vi "DAQ.Create.vi"(8 "error in":errorcluster, 11 "Instrument.DAQ":refnum<class "Instrument.DAQ.lvclass">) -> (0 "error out":errorcluster, 3 "Instrument.DAQ":refnum<class "Instrument.DAQ.lvclass">)   [LabVIEW 2019, in "Instrument.Lockin.lvlib" / "Instrument.DAQ.lvclass"]
uses:
  Instrument.DAQ.lvclass
  Instrument.DAQ.lvclass/Instrument.DAQ.ctl
  DAQmx/DAQmx.lvclass
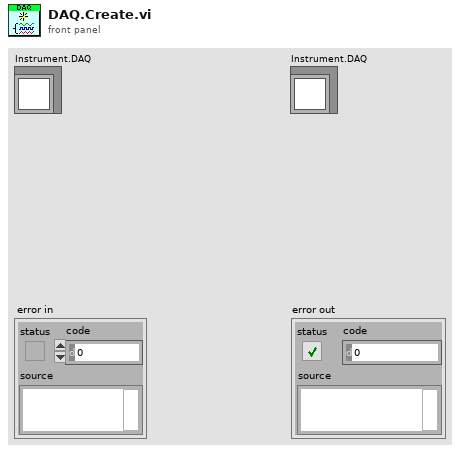
[diagram p1: front panel]
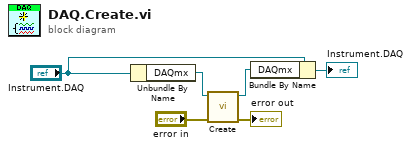
[diagram p0: block diagram]
diagram:
  n1 = Unbundle By Name("Instrument.DAQ") -> ("DAQmx"=w2:refnum<class "DAQmx.lvclass">)
  n2 = call "Create.vi"("error in"="error in", "DAQmx in"=w2) -> ("error out"=→"error out":errorcluster, "DAQmx out"=w1:refnum<class "DAQmx.lvclass">)  [unwired: 8 in]
  n3 = Bundle By Name(cluster="Instrument.DAQ", "DAQmx"=w1) -> (→"Instrument.DAQ":refnum<class "Instrument.DAQ.lvclass">)
